vi "Q2_Al_Arthur.vi"() -> ()   [LabVIEW 2019]
uses:
  <vilib>/measure/matone.llb/Extract Multiple Tone Information N Chan.vi
  <vilib>/measure/NI_MAPro.lvlib
panel:
  out "Potência Reativa":dbl
  out "Potência Ativa":dbl
  out "Potência aparente":dbl
  in  "Amplitude tensão 2":dbl format="%_6p"
  in  "Amplitude corrente 2":dbl format="%_6p"
  out "RESULTADO":string="Atinge a exigência"
  out "Fator de potência":dbl
  in  "detected phase":dbl format="%_6g"
  out "multiple tone information":T1(array[cluster]) {"multiple tone information"."detected phase (deg)" format="%_6g"; "multiple tone information"."detected amplitude" format="%_6p"; "multiple tone information"."detected frequency" format="%_6p"}
  out "Waveform Graph":waveform(dbl)[](graph)
  in  "file path":path
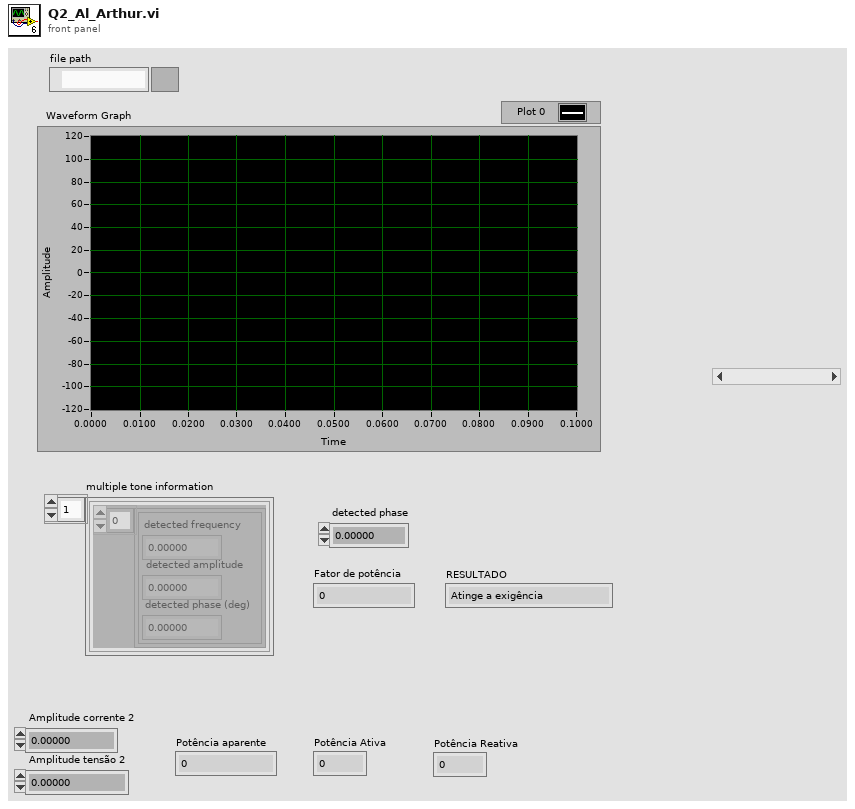
[diagram p1: front panel]
types:
  T1 = cluster{"multiple tone information":cluster{"detected frequency":dbl, "detected amplitude":dbl, "detected phase (deg)":dbl}[]}[]
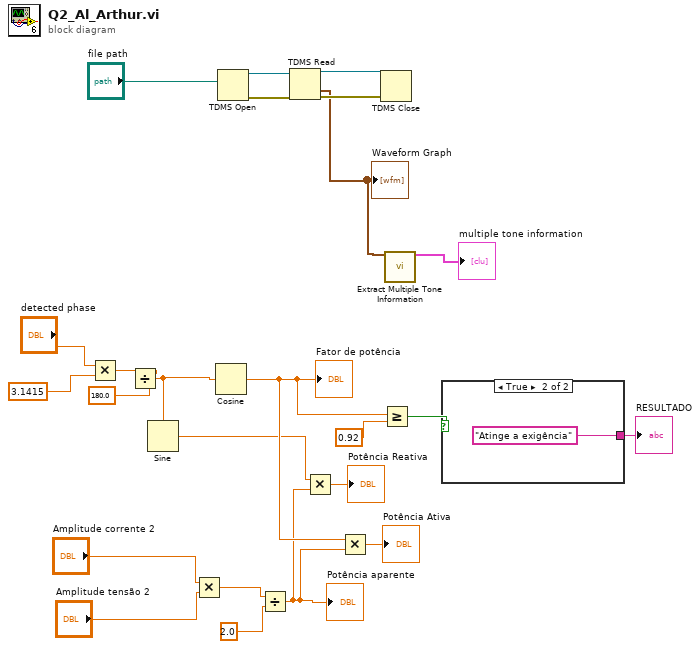
[diagram p0: block diagram]
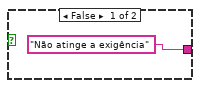
[diagram p2: hidden frame]
diagram:
  n1 = Multiply(x="detected phase", y=3.1415) -> (x*y=w15:dbl)
  n2 = Divide(x=w15, y=180.0) -> (x/y=w4:dbl)
  n3 = Sine(x=w4) -> (sin(x)=w2:dbl)
  n4 = Multiply(x="Amplitude corrente 2", y="Amplitude tensão 2") -> (x*y=w8:dbl)
  n5 = Cosine(x=w4) -> (cos(x)=w6:dbl)
  "Fator de potência" <- w6
  n6 = TDMS Open(11:"file path") -> (0:w23:errorcluster, 3:w24:refnum<k34>)  [unwired: 6 in]
  n7 = Divide(x=w8, y=2.0) -> (x/y=w3:dbl)
  "Potência aparente" <- w3
  n8 = TDMS Read(0:w24, 11:w23) -> (4:w22:refnum<k34>, 10:w19:waveform(dbl)[], 15:w21:errorcluster)  [unwired: 6 in, 3 out]
  "Waveform Graph" <- w19
  n9 = Multiply(x=w2, y=w3) -> (x*y=→"Potência Reativa":dbl)
  n10 = Multiply(x=w6, y=w3) -> (x*y=→"Potência Ativa":dbl)
  n11 = TDMS Close(8:w21, 11:w22) -> ()  [unwired: 2 out]
  n12 = Greater Or Equal?(x=w6, y=0.92) -> (x >= y?=w12:bool)
  n13 = call-poly <vilib>:"Extract Multiple Tone Information.vi"("time signals in"=w19) -> ("multiple tone information"=→"multiple tone information":T1)  [unwired: 12 in, 2 out]
  n14 = case shown="True" w12 {
    tunnel: ["Não atinge a exigência" "Atinge a exigência"] -> w11
    frame False {
    }
    frame True {
    }
  }
  "RESULTADO" <- w11
